vi "destroy.vi"(5 "timeout when waiting (10000ms)":u32=10000, 7 "Wait until all data is streamed? (T)":bool=TRUE, 8 "error in":errorcluster, 11 "stream custom cluster":refnum<class "stream_custom_cluster.lvclass">) -> (0 "error out":errorcluster)   [LabVIEW 2020, in "stream_custom_cluster.lvclass"]
doc: "Releases memory used by the buffering system.\nWhen \"Wait until all data is streamed\" is enabled, waits for buffer size = 0.\n10-second default timeout prevents indefinite waiting.\nSee `Streaming Cluster Data` example for useage notes."
uses:
  stream_custom_cluster.lvclass
  stream_custom_cluster.lvclass/stream_custom_cluster.ctl
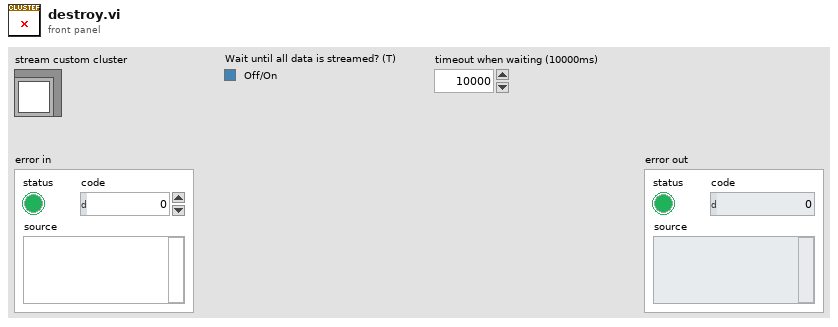
[diagram p1: front panel]
types:
  T1 = typedef "stream_custom_cluster.lvclass/private data.ctl" = cluster{"type":T2[], "channel names":string[], "data":refnum<queue>[], "cluster element types":variant[]}
  T2 = typedef "openg_variant.lvlib/Type Descriptor Enumeration__ogtk.ctl" = enum8{"<Null>", "I8", "I16", "I32", "I64", "U8", "U16", "U32", "U64", "SGL", "DBL", "EXT", "CSG", "CDB", "CXT", "0x0F", "0x10", "0x11", "0x12", "0x13", "0x14", "Enum U8", "Enum U16", "Enum U32", "Enum U64", "SGL PQ", "DBL PQ", "EXT PQ", "CSG PQ", "CDB PQ", "CXT PQ", "0x1F", "0x20", "Boolean", "0x22", "0x23", "0x24", "0x25", "0x26", "0x27", "0x28", "0x29", "0x2A", "0x2B", "0x2C", "0x2D", "0x2E", "0x2F", "String", "0x31", "Path", "Pict", "0x34", "0x35", "0x36", "DAQ", "0x38", "0x39", "0x3A", "0x3B", "0x3C", "0x3D", "0x3E", "0x3F", "Array", "0x41", "0x42", "0x43", "0x44", "0x45", "0x46", "0x47", "0x48", "0x49", "0x4A", "0x4B", "0x4C", "0x4D", "0x4E", "0x4F", "Cluster", "0x51", "0x52", "Variant", "Waveform", "0x55", "0x56", "0x57", "0x58", "0x59", "0x5A", "0x5B", "0x5C", "0x5D", "0x5E", "Fixed Point", "0x60", "0x61", "0x62", "0x63", "0x64", "0x65", "0x66", "0x67", "0x68", "0x69", "0x6A", "0x6B", "0x6C", "0x6D", "0x6E", "0x6F", "Refnum", "0x71", "0x72", "Set Collection", "Map Collection"}
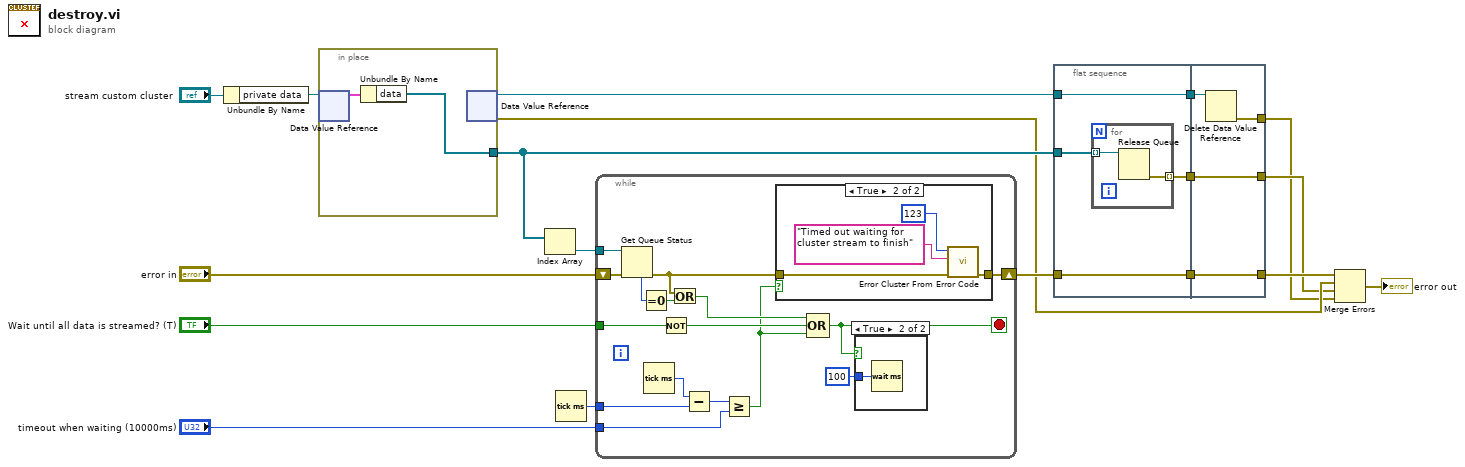
[diagram p0: block diagram]
diagram:
  n1 = Unbundle By Name("stream custom cluster") -> ("private data"=w17:refnum<data-value>)
  n2 = in-place {
    in-place-border: [w19] -> w10
    n3 = in-place-dvr #1(w17) -> (w20:T1)  [unwired: 1 out]
    n4 = Unbundle By Name(w20) -> ("data"=w19:refnum<queue>[])
    n5 = in-place-dvr #1() -> (w15:refnum<data-value>, w4:errorcluster)  [unwired: 1 in]
  }
  n6 = Index Array(array=w10) -> (element=w12:refnum<queue>)  [unwired: 1 in]
  n7 = Tick Count (ms)() -> (millisecond timer value=w7:u32)
  n8 = while {
    tunnel: w12 -> [w36]
    shift-right: [w22] -> w8
    shift-left: "error in" -> [w35]
    tunnel: "Wait until all data is streamed? (T)" -> [w26]
    tunnel: w7 -> [w31]
    tunnel: "timeout when waiting (10000ms)" -> [w28]
    stop <- w24 stop-if-true
    n9 = Get Queue Status(queue=w36, error in (no error)=w35) -> (error out=w23:errorcluster, # elements in queue=w34:i32)  [unwired: 1 in, 6 out]
    n10 = Equal To 0?(x=w34) -> (x = 0?=w33:bool)
    n11 = Tick Count (ms)() -> (millisecond timer value=w30:u32)
    n12 = Not(x=w26) -> (.not. x?=w25:bool)
    n13 = Or(x=w23, y=w33) -> (x .or. y?=w27:bool)
    n14 = Subtract(x=w30, y=w31) -> (x-y=w29:u32)
    n15 = Greater Or Equal?(x=w29, y=w28) -> (x >= y?=w21:bool)
    n16 = case shown="True" w21 {
      tunnel: w23 -> [w37 w40]
      tunnel: [w37 w39] -> w22
      frame False {
      }
      frame True {
        n17 = call <vilib>:"Error Cluster From Error Code.vi"("error in (no error)"=w40, "error message (\"\")"="Timed out waiting for cluster stream to finish" ("error message (\"\")"), "error code (0)"=123) -> ("error out"=w39:errorcluster)  [unwired: 6 in]
      }
    }
    n18 = Compound Arithmetic op=OR(w27, w25, w21) -> (w24:bool)
    n19 = case shown="True" w24 {
      tunnel: u32 100 -> [_ w42]
      frame False {
      }
      frame True {
        n20 = Wait (ms)(milliseconds to wait=w42) -> ()  [unwired: 1 out]
      }
    }
  }
  n21 = flat-sequence {
    tunnel: w15 -> [w46]
    tunnel: [w46] -> w11
    tunnel: w10 -> [w45]
    tunnel: [w44] -> w9
    tunnel: w8 -> [w44]
    tunnel: [w43] -> w2
    tunnel: w11 -> [w52]
    tunnel: [w51] -> w5
    tunnel: w9 -> [w51]
    tunnel: [w50] -> w3
    tunnel: w2 -> [w50]
    tunnel: [w49] -> w1
    frame #0 {
      n22 = for {
        tunnel: w45 -> [w48] mode=indexing
        tunnel: [w47] -> w43 mode=indexing
        n23 = Release Queue(queue=w48) -> (error out=w47:errorcluster)  [unwired: 2 in, 2 out]
      }
    }
    frame #1 {
      n24 = Delete Data Value Reference(data value reference=w52) -> (error out=w49:errorcluster)  [unwired: 1 in, 1 out]
    }
  }
  n25 = Merge Errors(w5, w4, w3, w1) -> (→"error out":errorcluster)
